vi "MCLB Request Edit Cell.vi"(8 "error in (no error)":errorcluster, 10 "Cell Position":T1, 11 "View in":refnum<class "Resource View.lvclass">) -> (0 "error out":errorcluster, 1 "Edited Cell":T1, 2 "Value":string, 3 "View out":refnum<class "Resource View.lvclass">, 5 "Modified?":bool)   [LabVIEW 2013, in "SET Project Editor.lvlib" / "Resource View.lvclass"]
uses:
  Resource View.lvclass
  <vilib>/Utility/miscctls.llb/LVRowAndColumnTypeDef.ctl
  MCListbox View/MCListbox View.lvclass
  <vilib>/ActorFramework/Actor/Actor.lvclass/Actor.ctl
  Resource View.lvclass/Resource View.ctl
  <vilib>/ActorFramework/Message Enqueuer/Message Enqueuer.lvclass/Message Enqueuer.ctl
  <vilib>/ActorFramework/Message Enqueuer/Enqueue.vi
  <vilib>/ActorFramework/Message Priority Queue/Priority Enqueue.vi
  Controller Messages/Set Modified Flag Msg/Set Modified Flag Msg.lvclass
  <vilib>/ActorFramework/Actor/Actor.lvclass
  SET Project Data/Resource Data Class/Resource Data.lvclass
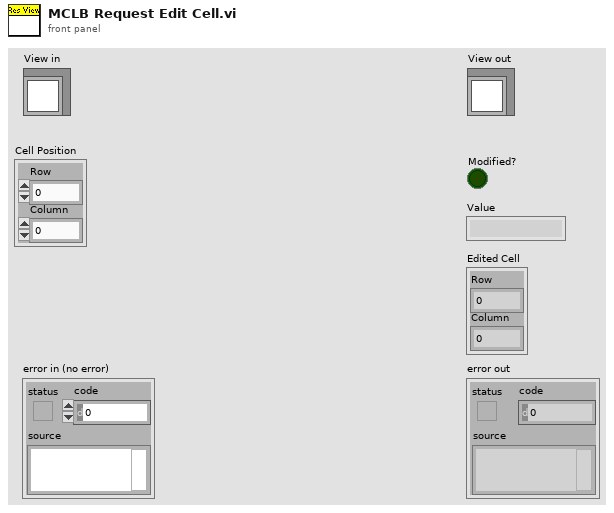
[diagram p1: front panel]
types:
  T1 = typedef "LVRowAndColumnTypeDef.ctl" = cluster{"Row":i32, "Column":i32}
  T2 = typedef "SET Project Data.lvlib/ProjFile_Resource Entry.ctl" = cluster{"RID":string, "Tag":string, "Strings [] (UTF-16)":string[], "Shared?":bool}
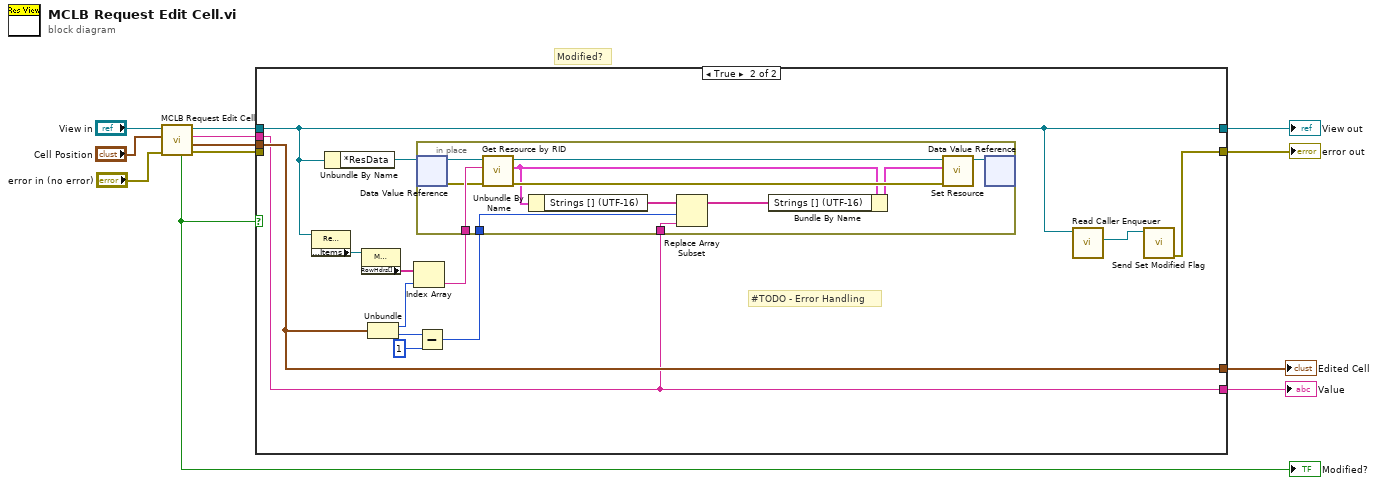
[diagram p0: block diagram]
diagram:
  # "Modified?"
  n1 = call-parent "MCLB Request Edit Cell.vi"("error in (no error)"="error in (no error)", "RowAndCollumn"="Cell Position", "View in"="View in") -> ("error out"=w9:errorcluster, "Edited Cell"=w6:T1, "Value"=w8:string, "View out"=w7:refnum<class "Resource View.lvclass">, "Modified?"=w1:bool)  [unwired: 4 in]
  "Modified?" <- w1
  n2 = case shown="True" w1 {
    tunnel: w9 -> [w15 _]
    tunnel: w8 -> [w14 w17]
    tunnel: w7 -> [w16 w20]
    tunnel: w6 -> [w13 w22]
    tunnel: [w15 w23] -> w5
    tunnel: [w16 w20] -> w4
    tunnel: [w13 w22] -> w3
    tunnel: [w14 w17] -> w2
    frame False {
    }
    frame True {
      # "#TODO - Error Handling"
      n3 = property class="Resource View.lvclass"(reference=w20) -> ("Properties:Items"=w25:refnum<vi>)  [unwired: 1 in, 2 out]
      n4 = Unbundle By Name(w20) -> ("*ResData"=w21:refnum<data-value>)
      n5 = property class="MCListbox"(reference=w25) -> ("RowHdrs[]"=w26:string[])  [unwired: 1 in, 2 out]
      n6 = Unbundle(w22) -> ("Row"=w27:i32, "Column"=w28:i32)
      n7 = Index Array(array=w26, index=w27) -> (element=w19:string)
      n8 = Subtract(x=w28, y=1) -> (x-y=w18:i32)
      n9 = in-place {
        in-place-border: w19 -> [w40]
        in-place-border: w18 -> [w34]
        in-place-border: w17 -> [w33]
        n10 = in-place-dvr #1(w21) -> (w41:refnum<class "Resource Data.lvclass">, w39:errorcluster)
        n11 = call "Get Resource by RID.vi"("error in (no error)"=w39, "RID"=w40, "LangFile in"=w41) -> ("error out"=w36:errorcluster, "Resource"=w32:T2, "LangFile out"=w38:refnum<class "Resource Data.lvclass">)  [unwired: 4 in, 2 out]
        n12 = Unbundle By Name(w32) -> ("Strings [] (UTF-16)"=w35:string[])
        n13 = Replace Array Subset(array=w35, new element=w33, index=w34) -> (w31:string[])
        n14 = Bundle By Name(cluster=w32, "Strings [] (UTF-16)"=w31) -> (w30:T2)
        n15 = call "Set Resource.vi"("error in (no error)"=w36, "Resource"=w30, "LangFile in"=w38) -> ("LangFile out"=w37:refnum<class "Resource Data.lvclass">)  [unwired: 7 in, 1 out]
        n16 = in-place-dvr #1(w37) -> ()  [unwired: 2 out]
      }
      n17 = call <vilib>:"Read Caller Enqueuer.vi"("Actor"=w20) -> ("Caller Enqueuer"=w24:refnum<class "Message Enqueuer.lvclass">)  [unwired: 10 in]
      n18 = call "Send Set Modified Flag.vi"("Message Enqueuer"=w24) -> ("error out"=w23:errorcluster)  [unwired: 9 in, 1 out]
    }
  }
  "error out" <- w5
  "View out" <- w4
  "Value" <- w2
  "Edited Cell" <- w3
